vi "SD-LV70TimeStampToDateRec.vi"(1 "time stamp":timestamp) -> (0 "date time rec":T1)   [LabVIEW 2020]
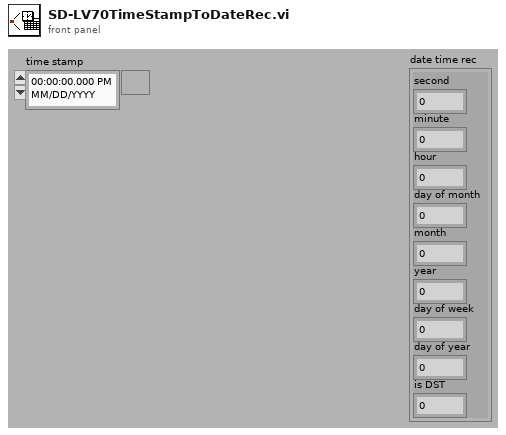
[diagram p1: front panel]
types:
  T1 = cluster{"second":i32, "minute":i32, "hour":i32, "day of month":i32, "month":i32, "year":i32, "day of week":i32, "day of year":i32, "is DST":i32}
  T2 = typedef "LVDateTimeRec.ctl" = cluster{"fractional second":dbl, "second":i32, "minute":i32, "hour":i32, "day of month":i32, "month":i32, "year":i32, "day of week":i32, "day of year":i32, "DST":i32}
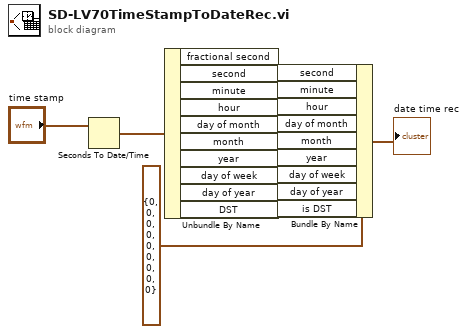
[diagram p0: block diagram]
diagram:
  n1 = Seconds To Date/Time(time stamp (now)="time stamp") -> (date time rec=w1:T2)  [unwired: 1 in]
  n2 = Unbundle By Name(w1) -> ("second"=w4:i32, "minute"=w5:i32, "hour"=w6:i32, "day of month"=w7:i32, "month"=w8:i32, "year"=w9:i32, "day of week"=w10:i32, "day of year"=w11:i32, "DST"=w12:i32)  [unwired: 1 out]
  n3 = Bundle By Name(cluster=T1 {"second"=0, "minute"=0, "hour"=0, "day of month"=0, "month"=0, "year"=0, "day of week"=0, "day of year"=0, "is DST"=0} ("date time rec"), "second"=w4, "minute"=w5, "hour"=w6, "day of month"=w7, "month"=w8, "year"=w9, "day of week"=w10, "day of year"=w11, "is DST"=w12) -> (→"date time rec":T1)
